vi "Teleop.vi"(10 "Match Info":T1={"Autonomous Elapsed Seconds"=0.0, "TeleOp Elapsed Seconds"=0.0, "Disabled Elapsed Seconds"=0.0, "Visited Autonomous"=FALSE, "Visited TeleOp"=FALSE, "Visited Disabled"=FALSE, "Autonomous Settings"={"Autonomous Style"=enum."Independent", "VI Refnum"=refnum}}, 11 "Call Context":T2) -> ()   [LabVIEW 2019]
doc: "This VI is called for each enabled TeleOp packet received from the DS. It is typically used to read from joysticks and other inputs and update I/O or setpoints for timed control loops. It should complete and return within 20 milliseconds or risk missing DS packets."
uses:
  <vilib>/Rock Robotics/WPI/DriverStation/WPI_DriverStationDerivedRobotMode.ctl
  <vilib>/Rock Robotics/WPI/DriverStation/WPI_DriverStationMatch Info.ctl
  <vilib>/Rock Robotics/WPI/Utilities/WPI_GetSetVariantRefNum.vi
  <vilib>/Rock Robotics/Network Tables/NT Write Boolean Array.vi
  <vilib>/Rock Robotics/Network Tables/NT Write Boolean.vi
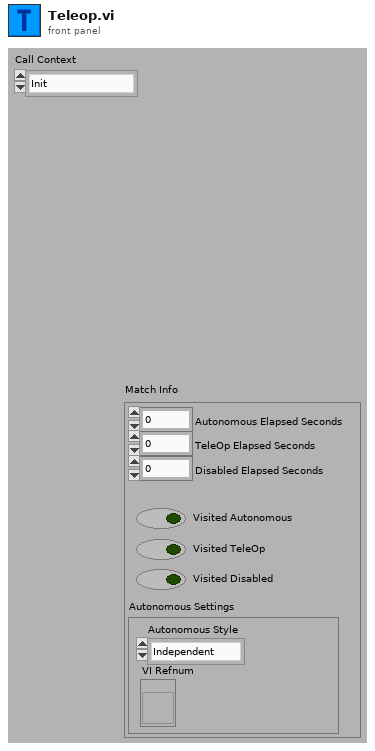
[diagram p1: front panel]
types:
  T1 = typedef "WPI_DriverStationMatch Info.ctl" = cluster{"Autonomous Elapsed Seconds":dbl, "TeleOp Elapsed Seconds":dbl, "Disabled Elapsed Seconds":dbl, "Visited Autonomous":bool, "Visited TeleOp":bool, "Visited Disabled":bool, "Autonomous Settings":cluster{"Autonomous Style":enum16{"Iterative", "Independent"}, "VI Refnum":refnum<vi>}}
  T2 = typedef "WPI_DriverStationDerivedRobotMode.ctl" = enum16{"Init", "Execute", "Stop"}
  T3 = enum16{"Low Ball", "Middle Ball", "High Ball", "High Hatch", "Middle Hatch", "Low Hatch", "Cargo Ball", "Ball Loading Station", "Ball Ground", "Reserve"}
  T4 = typedef "WPI_JoystickDevRef.ctl" = cluster{"Device":T5}
  T5 = typedef "WPI_JoystickDeviceEnum.ctl" = enum16{"USB 0", "USB 1", "USB 2", "USB 3", "USB 4", "USB 5"}
  T6 = cluster{"POVs[0]":i16, "POVs[1]":i16, "POVs[2]":i16, "POVs[3]":i16, "POVs[4]":i16, "POVs[5]":i16, "POVs[6]":i16, "POVs[7]":i16, "POVs[8]":i16}
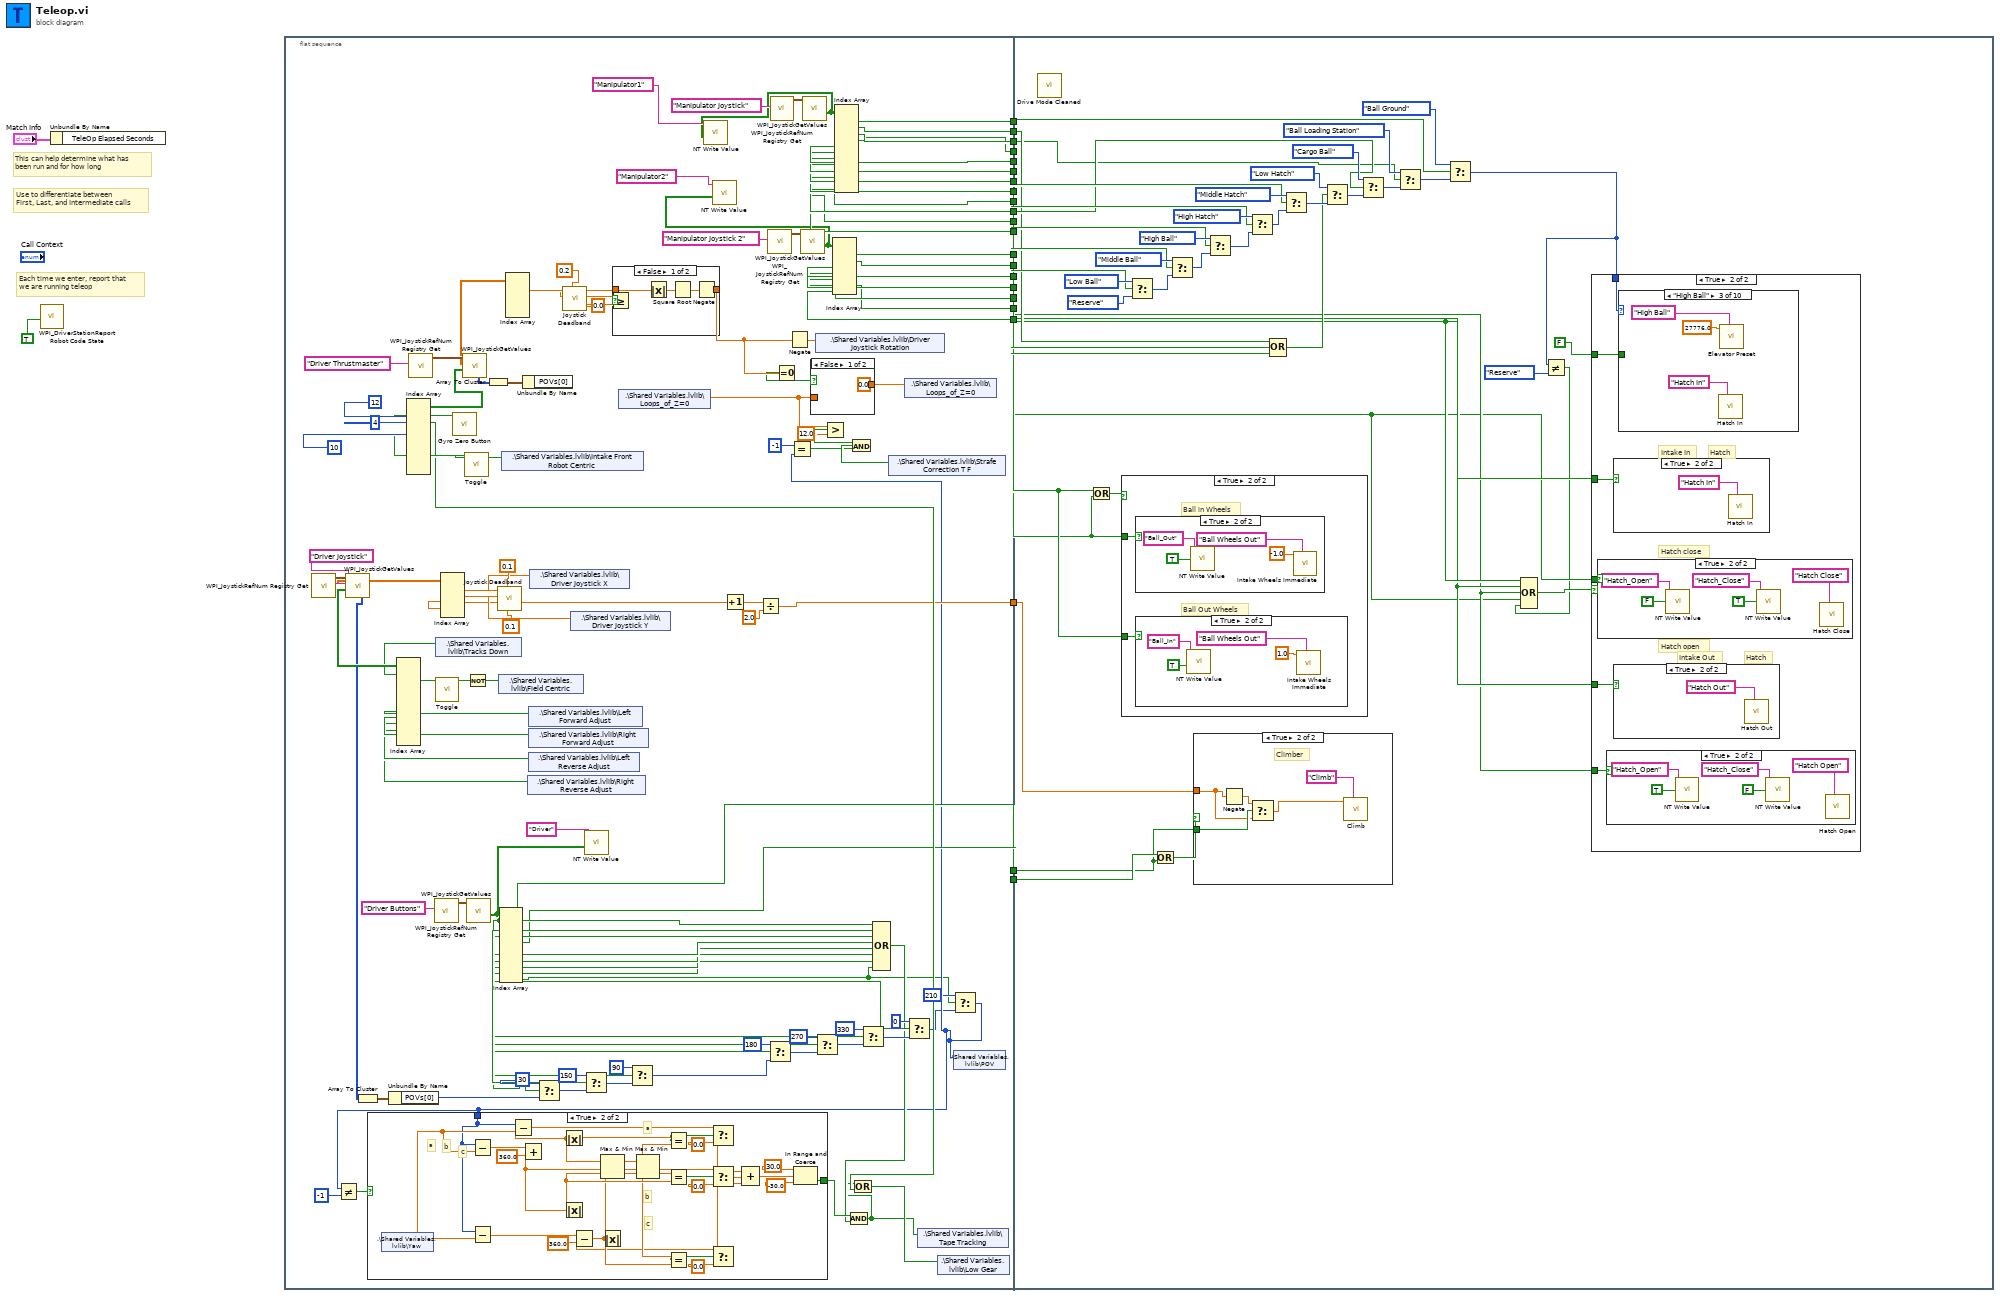
[diagram p0: block diagram]
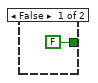
[diagram p2: hidden frame]
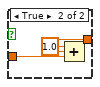
[diagram p3: hidden frame]
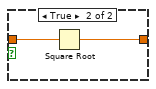
[diagram p4: hidden frame]
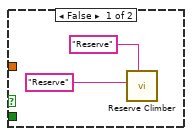
[diagram p5: hidden frame]
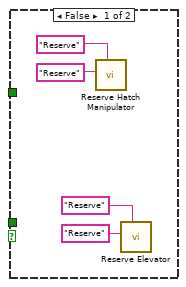
[diagram p6: hidden frame]
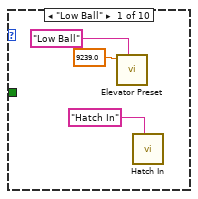
[diagram p7: hidden frame]
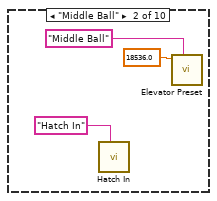
[diagram p8: hidden frame]
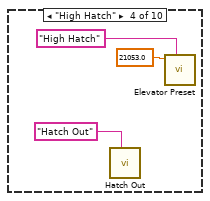
[diagram p9: hidden frame]
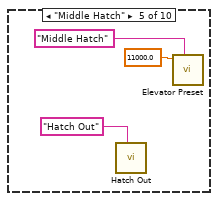
[diagram p10: hidden frame]
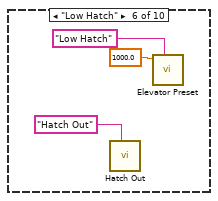
[diagram p11: hidden frame]
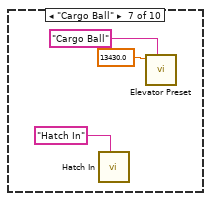
[diagram p12: hidden frame]
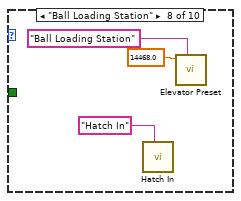
[diagram p13: hidden frame]
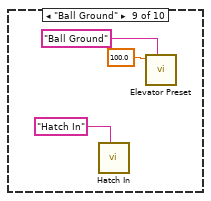
[diagram p14: hidden frame]
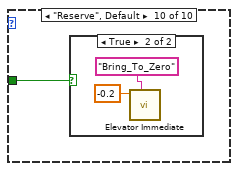
[diagram p15: hidden frame]
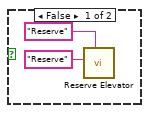
[diagram p16: hidden frame]
diagram:
  # "Each time we enter, report that\nwe are running teleop"
  # "Use to differentiate between\nFirst, Last, and Intermediate calls"
  # "This can help determine what has\nbeen run and for how long"
  n1 = call <vilib>:"WPI_DriverStationReport Robot Code State.vi"("TeleOp"=TRUE ("Autonomous")) -> ()  [unwired: 10 in, 1 out]
  n2 = Unbundle By Name("Match Info") -> ()  [unwired: 1 out]
  n3 = flat-sequence {
    tunnel: [w38] -> w22
    tunnel: [w99] -> w21
    tunnel: [w98] -> w20
    tunnel: [w97] -> w19
    tunnel: [w96] -> w18
    tunnel: [w95] -> w17
    tunnel: [w94] -> w16
    tunnel: [w93] -> w15
    tunnel: [w92] -> w14
    tunnel: [w91] -> w13
    tunnel: [w90] -> w12
    tunnel: [w89] -> w11
    tunnel: [w88] -> w10
    tunnel: [w87] -> w9
    tunnel: [w86] -> w8
    tunnel: [w85] -> w7
    tunnel: [w84] -> w6
    tunnel: [w83] -> w5
    tunnel: [w82] -> w4
    tunnel: [w81] -> w3
    tunnel: [w43] -> w2
    tunnel: [w42] -> w1
    tunnel: w22 -> [w182]
    tunnel: w21 -> [w198]
    tunnel: w20 -> [w201]
    tunnel: w19 -> [w197]
    tunnel: w18 -> [w203]
    tunnel: w17 -> [w200]
    tunnel: w16 -> [w206]
    tunnel: w15 -> [w204]
    tunnel: w14 -> [w193]
    tunnel: w13 -> [w207]
    tunnel: w12 -> [w202]
    tunnel: w11 -> [w205]
    tunnel: w10 -> [w194]
    tunnel: w9 -> [w189]
    tunnel: w8 -> [_]
    tunnel: w7 -> [w192]
    tunnel: w6 -> [w190]
    tunnel: w5 -> [w191]
    tunnel: w4 -> [_]
    tunnel: w3 -> [w196]
    tunnel: w2 -> [w184]
    tunnel: w1 -> [w183]
    frame #0 {
      n4 = call <vilib>:"WPI_JoystickRefNum Registry Get.vi"("refnum name"="Driver Joystick") -> ("JoystickDevRef"=w141:T4)  [unwired: 1 in, 9 out]
      n5 = call <vilib>:"WPI_JoystickGetValues.vi"("JoystickDevRef"=w141) -> ("Buttons"=w127:bool[], "Axes"=w139:dbl[], "POVs"=w114:i16[])  [unwired: 6 in, 2 out]
      n6 = Array To Cluster(array=w114) -> (cluster=w115:T6)
      n7 = Unbundle By Name(w115) -> ("POVs[0]"=w77:i16)
      n8 = Index Array(array=w127) -> (element #1=w102:bool, element #2=w101:bool, element #7=w112:bool, element #8=w111:bool, element #9=w110:bool, element #10=w109:bool)  [unwired: 12 in, 6 out]
      n9 = call <vilib>:"WPI_JoystickRefNum Registry Get.vi"("refnum name"="Driver Thrustmaster") -> ("JoystickDevRef"=w129:T4)  [unwired: 9 in, 1 out]
      n10 = call <vilib>:"WPI_JoystickRefNum Registry Get.vi"("refnum name"="Driver Buttons") -> ("JoystickDevRef"=w79:T4)  [unwired: 1 in, 9 out]
      n11 = shared-variable ".\\Shared Variables.lvlib\\Tracks Down"(w102) -> ()  [unwired: 1 in, 1 out]
      n12 = call "Toggle.vi"("Input"=w101) -> ("Output"=w134:bool)  [unwired: 9 in, 1 out]
      n13 = Index Array(array=w139) -> (element #1=w133:dbl, element #2=w132:dbl, element #4=w103:dbl)  [unwired: 5 in, 2 out]
      n14 = call <vilib>:"WPI_JoystickGetValues.vi"("JoystickDevRef"=w129) -> ("Buttons"=w124:bool[], "Axes"=w128:dbl[], "POVs"=w116:i16[])  [unwired: 6 in, 2 out]
      n15 = Index Array(array=w124, index #1=12 ("index"), index #2=4 ("index"), index #4=10 ("index")) -> (element #1=w122:bool, element #2=w46:bool, element #4=w117:bool)  [unwired: 7 in, 7 out]
      n16 = call "Gyro Zero Button.vi"("Boolean"=w122) -> ()  [unwired: 11 in]
      n17 = call "Toggle.vi"("Input"=w117) -> ("Output"=w118:bool)  [unwired: 9 in, 1 out]
      n18 = Not(x=w134) -> (.not. x?=w131:bool)
      n19 = call <vilib>:"WPI_JoystickGetValues.vi"("JoystickDevRef"=w79) -> ("Buttons"=w36:bool[])  [unwired: 6 in, 4 out]
      n20 = Array To Cluster(array=w116) -> (cluster=w120:T6)
      n21 = call "Joystick Deadband.vi"("Z Deadband"=0.1, "X Y Deadband"=0.1, "Z"=w103, "Y"=w132, "X"=w133) -> ("Z Out"=w41:dbl, "Y Out"=w135:dbl, "X Out"=w107:dbl)  [unwired: 4 in]
      n22 = shared-variable ".\\Shared Variables.lvlib\\Field Centric"(w131) -> ()  [unwired: 1 in, 1 out]
      n23 = Index Array(array=w36) -> (element #1=w58:bool, element #2=w64:bool, element #3=w63:bool, element #4=w43:bool, element #5=w42:bool, element #6=w62:bool, element #7=w61:bool, element #8=w60:bool, element #9=w59:bool, element #10=w25:bool)  [unwired: 10 in]
      n24 = shared-variable ".\\Shared Variables.lvlib\\Intake Front Robot Centric"(w118) -> ()  [unwired: 1 in, 1 out]
      n25 = Index Array(array=w128) -> (element #1=w106:dbl)  [unwired: 5 in, 4 out]
      n26 = Unbundle By Name(w120) -> ()  [unwired: 1 out]
      n27 = shared-variable ".\\Shared Variables.lvlib\\Right Reverse Adjust"(w109) -> ()  [unwired: 1 in, 1 out]
      n28 = shared-variable ".\\Shared Variables.lvlib\\Left Forward Adjust"(w112) -> ()  [unwired: 1 in, 1 out]
      n29 = shared-variable ".\\Shared Variables.lvlib\\Right Forward Adjust"(w111) -> ()  [unwired: 1 in, 1 out]
      n30 = shared-variable ".\\Shared Variables.lvlib\\Left Reverse Adjust"(w110) -> ()  [unwired: 1 in, 1 out]
      n31 = shared-variable ".\\Shared Variables.lvlib\\Driver Joystick X"(w107) -> ()  [unwired: 1 in, 1 out]
      n32 = Select(t=i16 30, s=w58, f=w77) -> (s? t:f=w72:i16)
      n33 = call "Joystick Deadband.vi"("X Y Deadband"=0.2, "X"=w106) -> ("X Out"=w104:dbl)  [unwired: 7 in, 2 out]
      n34 = shared-variable ".\\Shared Variables.lvlib\\Driver Joystick Y"(w135) -> ()  [unwired: 1 in, 1 out]
      n35 = Select(t=i16 150, s=w64, f=w72) -> (s? t:f=w71:i16)
      n36 = call-poly <vilib>:"NT Write Value.vi"("Boolean Array"=w36, "Name"="Driver") -> ()  [unwired: 9 in, 1 out]
      n37 = Greater Or Equal?(x=w104, y=0.0) -> (x >= y?=w126:bool)
      n38 = case shown="False" w126 {
        tunnel: [w175 w179] -> w54
        tunnel: w104 -> [w174 w178]
        frame False {
          n39 = Absolute Value(x=w174) -> (abs(x)=w177:dbl)
          n40 = Square Root(x=w177) -> (sqrt(x)=w176:dbl)
          n41 = Negate(x=w176) -> (-x=w175:dbl)
        }
        frame True {
          n42 = Square Root(x=w178) -> (sqrt(x)=w179:dbl)
        }
      }
      n43 = shared-variable ".\\Shared Variables.lvlib\\Loops_of_Z=0"() -> (w50:dbl)  [unwired: 1 in, 1 out]
      n44 = Select(t=i16 90, s=w63, f=w71) -> (s? t:f=w37:i16)
      n45 = Increment(x=w41) -> (x+1=w40:dbl)
      n46 = Divide(x=w40, y=2.0) -> (x/y=w38:dbl)
      n47 = call <vilib>:"WPI_JoystickRefNum Registry Get.vi"("refnum name"="Manipulator Joystick 2") -> ("JoystickDevRef"=w80:T4)  [unwired: 1 in, 9 out]
      n48 = Select(t=i16 180, s=w62, f=w37) -> (s? t:f=w69:i16)
      n49 = call <vilib>:"WPI_JoystickRefNum Registry Get.vi"("refnum name"="Manipulator Joystick") -> ("JoystickDevRef"=w137:T4)  [unwired: 1 in, 9 out]
      n50 = Equal To 0?(x=w54) -> (x = 0?=w53:bool)
      n51 = Negate(x=w54) -> (-x=w108:dbl)
      n52 = call <vilib>:"WPI_JoystickGetValues.vi"("JoystickDevRef"=w80) -> ("Buttons"=w31:bool[])  [unwired: 6 in, 4 out]
      n53 = call-poly <vilib>:"NT Write Value.vi"("Boolean Array"=w31, "Name"="Manipulator2") -> ()  [unwired: 9 in, 1 out]
      n54 = call <vilib>:"WPI_JoystickGetValues.vi"("JoystickDevRef"=w137) -> ("Buttons"=w32:bool[])  [unwired: 6 in, 4 out]
      n55 = call-poly <vilib>:"NT Write Value.vi"("Boolean Array"=w32, "Name"="Manipulator1") -> ()  [unwired: 9 in, 1 out]
      n56 = case shown="False" w53 {
        tunnel: w50 -> [_ w173]
        tunnel: [0.0 w171] -> w52
        frame False {
        }
        frame True {
          n57 = Add(x=1.0, y=w173) -> (x+y=w171:dbl)
        }
      }
      n58 = Select(t=i16 270, s=w61, f=w69) -> (s? t:f=w67:i16)
      n59 = shared-variable ".\\Shared Variables.lvlib\\Driver Joystick Rotation"(w108) -> ()  [unwired: 1 in, 1 out]
      n60 = Greater?(x=w50, y=12.0) -> (0:w51:bool)
      n61 = Index Array(array=w31) -> (element #1=w87:bool, element #2=w86:bool, element #3=w85:bool, element #4=w84:bool, element #5=w83:bool, element #6=w82:bool, element #7=w81:bool)  [unwired: 7 in]
      n62 = Index Array(array=w32) -> (element #1=w99:bool, element #2=w98:bool, element #3=w97:bool, element #4=w96:bool, element #5=w95:bool, element #6=w94:bool, element #7=w93:bool, element #8=w92:bool, element #9=w91:bool, element #10=w90:bool, element #11=w89:bool, element #12=w88:bool)  [unwired: 12 in]
      n63 = Select(t=i16 330, s=w60, f=w67) -> (s? t:f=w65:i16)
      n64 = Compound Arithmetic op=OR(w58, w64, w63, w62, w61, w60, w59, w25) -> (w47:bool)
      n65 = shared-variable ".\\Shared Variables.lvlib\\Loops_of_Z=0"(w52) -> ()  [unwired: 1 in, 1 out]
      n66 = Select(t=i16 0, s=w59, f=w65) -> (s? t:f=w27:i16)
      n67 = Select(t=i16 210, s=w25, f=w27) -> (s? t:f=w28:i16)
      n68 = Not Equal?(x=w28, y=i16 -1) -> (x != y?=w30:bool)
      n69 = case shown="True" w30 {
        tunnel: [FALSE w167] -> w48
        tunnel: w28 -> [_ w144]
        frame False {
        }
        frame True {
          # "c"
          # "b"
          # "a"
          # "c"
          # "b"
          # "a"
          n70 = shared-variable ".\\Shared Variables.lvlib\\Yaw"() -> (w145:dbl)  [unwired: 1 in, 1 out]
          n71 = Subtract(x=w144, y=w145) -> (x-y=w166:dbl)
          n72 = Subtract(x=w144, y=w145) -> (x-y=w164:dbl)
          n73 = Subtract(x=w144, y=w145) -> (x-y=w155:dbl)
          n74 = Add(x=w166, y=360.0) -> (x+y=w156:dbl)
          n75 = Absolute Value(x=w155) -> (abs(x)=w161:dbl)
          n76 = Absolute Value(x=w156) -> (abs(x)=w160:dbl)
          n77 = Subtract(x=w164, y=360.0) -> (x-y=w154:dbl)
          n78 = Max & Min(x=w161, y=w160) -> (min(x,y)=w162:dbl)  [unwired: 1 out]
          n79 = Absolute Value(x=w154) -> (abs(x)=w158:dbl)
          n80 = Max & Min(x=w162, y=w158) -> (min(x,y)=w159:dbl)  [unwired: 1 out]
          n81 = Equal?(x=w161, y=w159) -> (x = y?=w153:bool)
          n82 = Equal?(x=w159, y=w160) -> (x = y?=w157:bool)
          n83 = Equal?(x=w159, y=w158) -> (x = y?=w152:bool)
          n84 = Select(t=w155, s=w153, f=0.0) -> (s? t:f=w148:dbl)
          n85 = Select(t=w156, s=w157, f=0.0) -> (s? t:f=w147:dbl)
          n86 = Select(t=w154, s=w152, f=0.0) -> (s? t:f=w146:dbl)
          n87 = Compound Arithmetic op=ADD(w148, w147, w146) -> (w143:dbl)
          n88 = In Range and Coerce(upper limit=30.0, x=w143, lower limit=-30.0) -> (In Range?=w167:bool)  [unwired: 1 out]
        }
      }
      n89 = Equal?(x=i16 -1, y=w28) -> (x = y?=w55:bool)
      n90 = And(x=w51, y=w55) -> (x .and. y?=w56:bool)
      n91 = Compound Arithmetic op=AND(w48, w47) -> (w44:bool)
      n92 = Or(x=w44, y=w46) -> (x .or. y?=w45:bool)
      n93 = shared-variable ".\\Shared Variables.lvlib\\Strafe Correction T F"(w56) -> ()  [unwired: 1 in, 1 out]
      n94 = shared-variable ".\\Shared Variables.lvlib\\Tape Tracking"(w44) -> ()  [unwired: 1 in, 1 out]
      n95 = shared-variable ".\\Shared Variables.lvlib\\Low Gear"(w45) -> ()  [unwired: 1 in, 1 out]
      n96 = shared-variable ".\\Shared Variables.lvlib\\POV"(w28) -> ()  [unwired: 1 in, 1 out]
    }
    frame #1 {
      # "Climber"
      n97 = call "Drive Mode Cleaned.vi"() -> ()  [unwired: 12 in]
      n98 = Or(x=w194, y=w193) -> (x .or. y?=w195:bool)
      n99 = case shown="True" w195 {
        tunnel: w194 -> [_ w294]
        tunnel: w193 -> [_ w293]
        frame False {
          n100 = call-poly <vilib>:"NT Write Value.vi"("Boolean"=FALSE, "Name"="Ball_Out") -> ()  [unwired: 9 in, 1 out]
          n101 = call "Reserve Intake.vi"("Description"="Reserve", "Command Name"="Reserve") -> ()  [unwired: 9 in, 1 out]
          n102 = call-poly <vilib>:"NT Write Value.vi"("Boolean"=FALSE, "Name"="Ball_In") -> ()  [unwired: 9 in, 1 out]
        }
        frame True {
          # "Ball in Wheels"
          # "Ball Out Wheels"
          n103 = case shown="True" w293 {
            frame False {
            }
            frame True {
              n104 = call-poly <vilib>:"NT Write Value.vi"("Boolean"=TRUE, "Name"="Ball_Out") -> ()  [unwired: 9 in, 1 out]
              n105 = call "Intake Wheels Immediate.vi"("Description"="Ball Wheels Out", "Setpoint"=-1.0) -> ()  [unwired: 9 in, 1 out]
            }
          }
          n106 = case shown="True" w294 {
            frame False {
            }
            frame True {
              n107 = call-poly <vilib>:"NT Write Value.vi"("Boolean"=TRUE, "Name"="Ball_In") -> ()  [unwired: 9 in, 1 out]
              n108 = call "Intake Wheels Immediate.vi"("Description"="Ball Wheels Out", "Setpoint"=1.0) -> ()  [unwired: 9 in, 1 out]
            }
          }
        }
      }
      n109 = Select(t=T3."Low Ball" ("Enum"), s=w203, f=T3."Reserve" ("Enum")) -> (s? t:f=w225:T3)
      n110 = Or(x=w184, y=w183) -> (x .or. y?=w185:bool)
      n111 = Select(t=T3."Middle Ball" ("Enum"), s=w204, f=w225) -> (s? t:f=w224:T3)
      n112 = case shown="True" w185 {
        tunnel: w183 -> [_ w231]
        tunnel: w182 -> [_ w229]
        frame False {
          n113 = call "Reserve Climber.vi"("Description"="Reserve", "Command Name"="Reserve" ("Description")) -> ()  [unwired: 9 in, 1 out]
        }
        frame True {
          n114 = Negate(x=w229) -> (-x=w230:dbl)
          n115 = Select(t=w230, s=w231, f=w229) -> (s? t:f=w228:dbl)
          n116 = call "Climb.vi"("Description"="Climb", "Setpoint"=w228) -> ()  [unwired: 9 in, 1 out]
        }
      }
      n117 = Select(t=T3."High Ball" ("Enum"), s=w205, f=w224) -> (s? t:f=w223:T3)
      n118 = Select(t=T3."High Hatch" ("Enum"), s=w207, f=w223) -> (s? t:f=w222:T3)
      n119 = Compound Arithmetic op=OR(w201, w200, w196) -> (w199:bool)
      n120 = Select(t=T3."Middle Hatch" ("Enum"), s=w206, f=w222) -> (s? t:f=w221:T3)
      n121 = Select(t=T3."Low Hatch" ("Enum"), s=w199, f=w221) -> (s? t:f=w220:T3)
      n122 = Select(t=T3."Cargo Ball" ("Enum"), s=w202, f=w220) -> (s? t:f=w219:T3)
      n123 = Select(t=T3."Ball Loading Station" ("Enum"), s=w197, f=w219) -> (s? t:f=w209:T3)
      n124 = Select(t=T3."Ball Ground" ("Enum"), s=w198, f=w209) -> (s? t:f=w187:T3)
      n125 = Not Equal?(x=w187, y=T3."Reserve" ("Enum")) -> (x != y?=w181:bool)
      n126 = Compound Arithmetic op=OR(w192, w191, w190, w189, w181) -> (w188:bool)
      n127 = case shown="True" w188 {
        tunnel: w192 -> [_ w242]
        tunnel: w190 -> [_ w241]
        tunnel: w191 -> [_ w240]
        tunnel: w189 -> [_ w239]
        tunnel: w187 -> [_ w238]
        tunnel: FALSE -> [_ w237]
        frame False {
          n128 = call "Reserve Hatch Manipulator.vi"("Description"="Reserve", "Command Name"="Reserve") -> ()  [unwired: 9 in, 1 out]
          n129 = call "Reserve Elevator.vi"("Description"="Reserve", "Command Name"="Reserve") -> ()  [unwired: 9 in, 1 out]
        }
        frame True {
          # "Hatch"
          # "Hatch"
          # "Hatch open"
          # "Hatch close"
          # "Intake In"
          # "Intake Out"
          n130 = case shown="True" w239 {
            frame False {
            }
            frame True {
              n131 = call-poly <vilib>:"NT Write Value.vi"("Boolean"=FALSE, "Name"="Hatch_Open") -> ()  [unwired: 9 in, 1 out]
              n132 = call-poly <vilib>:"NT Write Value.vi"("Boolean"=TRUE, "Name"="Hatch_Close") -> ()  [unwired: 9 in, 1 out]
              n133 = call "Hatch Close.vi"("Description"="Hatch Close") -> ()  [unwired: 10 in, 1 out]
            }
          }
          n134 = case shown="True" w241 {
            frame False {
            }
            frame True {
              n135 = call-poly <vilib>:"NT Write Value.vi"("Boolean"=TRUE, "Name"="Hatch_Open") -> ()  [unwired: 9 in, 1 out]
              n136 = call-poly <vilib>:"NT Write Value.vi"("Boolean"=FALSE, "Name"="Hatch_Close") -> ()  [unwired: 9 in, 1 out]
              n137 = call "Hatch Open.vi"("Description"="Hatch Open") -> ()  [unwired: 10 in, 1 out]
            }
          }
          n138 = case shown="True" w242 {
            frame False {
            }
            frame True {
              n139 = call "Hatch In.vi"("Description"="Hatch In") -> ()  [unwired: 10 in, 1 out]
            }
          }
          n140 = case shown="True" w240 {
            frame False {
            }
            frame True {
              n141 = call "Hatch Out.vi"("Description"="Hatch Out") -> ()  [unwired: 10 in, 1 out]
            }
          }
          n142 = case shown="\"High Ball\"" w238 {
            tunnel: w237 -> [_ _ _ _ _ _ _ _ _ w270]
            frame "Low Ball" {
              n143 = call "Elevator Preset.vi"("Description"="Low Ball", "Position"=9239.0) -> ()  [unwired: 9 in, 1 out]
              n144 = call "Hatch In.vi"("Description"="Hatch In") -> ()  [unwired: 10 in, 1 out]
            }
            frame "Middle Ball" {
              n145 = call "Hatch In.vi"("Description"="Hatch In") -> ()  [unwired: 10 in, 1 out]
              n146 = call "Elevator Preset.vi"("Description"="Middle Ball", "Position"=18536.0) -> ()  [unwired: 9 in, 1 out]
            }
            frame "High Ball" {
              n147 = call "Hatch In.vi"("Description"="Hatch In") -> ()  [unwired: 10 in, 1 out]
              n148 = call "Elevator Preset.vi"("Description"="High Ball", "Position"=27776.0) -> ()  [unwired: 9 in, 1 out]
            }
            frame "High Hatch" {
              n149 = call "Hatch Out.vi"("Description"="Hatch Out") -> ()  [unwired: 10 in, 1 out]
              n150 = call "Elevator Preset.vi"("Description"="High Hatch", "Position"=21053.0) -> ()  [unwired: 9 in, 1 out]
            }
            frame "Middle Hatch" {
              n151 = call "Hatch Out.vi"("Description"="Hatch Out") -> ()  [unwired: 10 in, 1 out]
              n152 = call "Elevator Preset.vi"("Description"="Middle Hatch", "Position"=11000.0) -> ()  [unwired: 9 in, 1 out]
            }
            frame "Low Hatch" {
              n153 = call "Hatch Out.vi"("Description"="Hatch Out") -> ()  [unwired: 10 in, 1 out]
              n154 = call "Elevator Preset.vi"("Description"="Low Hatch", "Position"=1000.0) -> ()  [unwired: 9 in, 1 out]
            }
            frame "Cargo Ball" {
              n155 = call "Hatch In.vi"("Description"="Hatch In") -> ()  [unwired: 10 in, 1 out]
              n156 = call "Elevator Preset.vi"("Description"="Cargo Ball", "Position"=13430.0) -> ()  [unwired: 9 in, 1 out]
            }
            frame "Ball Loading Station" {
              n157 = call "Hatch In.vi"("Description"="Hatch In") -> ()  [unwired: 10 in, 1 out]
              n158 = call "Elevator Preset.vi"("Description"="Ball Loading Station", "Position"=14468.0) -> ()  [unwired: 9 in, 1 out]
            }
            frame "Ball Ground" {
              n159 = call "Hatch In.vi"("Description"="Hatch In") -> ()  [unwired: 10 in, 1 out]
              n160 = call "Elevator Preset.vi"("Description"="Ball Ground", "Position"=100.0) -> ()  [unwired: 9 in, 1 out]
            }
            frame "Reserve", Default {
              n161 = case shown="True" w270 {
                frame False {
                  n162 = call "Reserve Elevator.vi"("Description"="Reserve", "Command Name"="Reserve") -> ()  [unwired: 9 in, 1 out]
                }
                frame True {
                  n163 = call "Elevator Immediate.vi"("Description"="Bring_To_Zero", "Speed"=-0.2) -> ()  [unwired: 9 in, 1 out]
                }
              }
            }
          }
        }
      }
    }
  }
